vi "Read Multi Value as Binary.vi"(6 "byte order":T1(ring), 8 "error in (no error)":errorcluster, 10 "Tag":string[](array[string]), 11 "Var Bus in":refnum<class "Omni_Bus.lvclass">) -> (0 "error out":errorcluster, 2 "Binary":string[](array[string]), 3 "Var Bus out":refnum<class "Omni_Bus.lvclass">)   [LabVIEW 2021, in "Omni_Bus.lvclass"]
uses:
  Omni_Bus.lvclass
  <vilib>/TSA/Abstract Data Classes/Abs_Types/Value/Abs_Value.lvclass
  Omni_Bus.lvclass/Omni_Bus.ctl
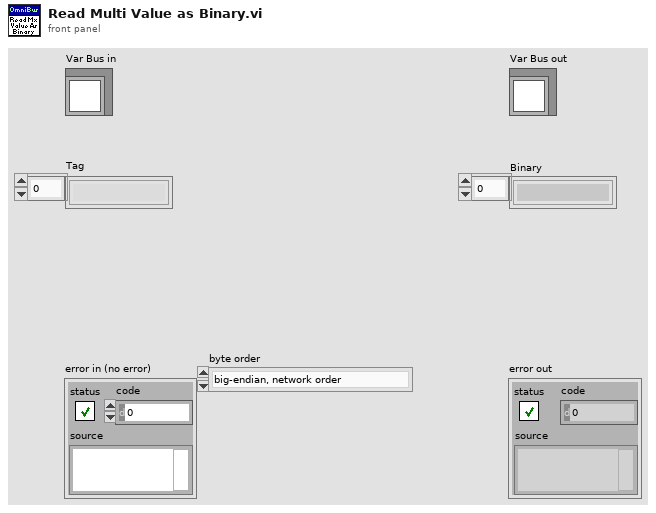
[diagram p1: front panel]
types:
  T1 = enum16{"big-endian, network order", "native, host order", "little-endian"}
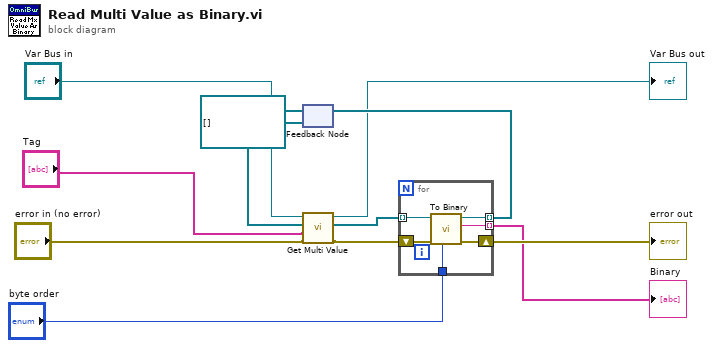
[diagram p0: block diagram]
diagram:
  n1 = feedback #1(refnum<class "Abs_Value.lvclass">[] []) -> (w5:refnum<class "Abs_Value.lvclass">[])
  n2 = call-dynamic "Get Multi Value.vi"("error in (no error)"="error in (no error)", "Tag"="Tag", "Value Type"=w5, "Var Bus in"="Var Bus in") -> ("error out"=w9:errorcluster, "Value Out"=w8:refnum<class "Abs_Value.lvclass">[], "Var Bus out"=→"Var Bus out":refnum<class "Omni_Bus.lvclass">)  [unwired: 5 in]
  n3 = for {
    tunnel: [w17] -> w11 mode=indexing
    tunnel: [w16] -> w10 mode=indexing
    tunnel: w8 -> [w14] mode=indexing
    tunnel: "byte order" -> [w13]
    shift-right: [w18] -> w12
    shift-left: w9 -> [w15]
    n4 = call-dynamic "To Binary.vi"("byte order"=w13, "error in (no error)"=w15, "Type in"=w14) -> ("error out"=w18:errorcluster, "Binary"=w17:string, "Type out"=w16:refnum<class "Abs_Value.lvclass">)  [unwired: 6 in]
  }
  "error out" <- w12
  "Binary" <- w11
  n5 = feedback-in #1(w10) -> ()
